vi "E709_All_VIs.vi"   [LabVIEW 2014, in "PiFOC.lvlib"]
doc: "This VI contains all high level and low level VIs valid for E-709. \nSee diagram for a survey of all E-709 high level and low level VIs. \nMenu / Browse / Show VI Hierarchy will show the file paths of the VIs. \nGlobal Variables are shown as Control as well as Indicator."
uses:
  PiFOC.lvlib
  Low Level/General command.llb/Controller names.ctl
  Low Level/Communication.llb/Available DLL interfaces.ctl
  Low Level/Communication.llb/Available DLLs.ctl
  Low Level/Communication.llb/Available interfaces.ctl
  Low Level/Communication.llb/Termination character.ctl
  Low Level/Analog control.llb/Available Analog Commands.ctl
  Low Level/Communication.llb/Global1.vi
  Low Level/General command.llb/Global2 (Array).vi
  Low Level/Communication.llb/Global DaisyChain.vi
  Low Level/Analog control.llb/Global Analog.vi
  Low Level/Support.llb/Unbunde/bundle interface clusters for PI Terminal.vi
panel:
  # "E-709 PI GCS LabVIEW driver set"
  # "This VI contains all high level and low level VIs valid for E-709. See diagram for a survey of all E-709 high \nlevel and low level VIs. Menu / Browse / Show VI Hierarchy will show the file paths of the VIs. Global \nVariables are shown as Control as well as Indicator."
types:
  T1 = typedef "PiFOC.lvlib/Available Analog Commands.ctl" = enum16{"INITIALIZE", "VOL?", "VOL ", "CLOSE", "MOV", "POS?", "VCO", "VCO?", "WAIT_WF", "TMN?", "TMX?", "VEL", "VEL?", "SAI?", "MVR", "ERR?", "#24", "STP", "*IDN?", "#5", "STE", "DRR?", "W_Wave", "HLP?", "W/R_Wave"}
  T2 = typedef "PiFOC.lvlib/Termination character.ctl" = enum16{"LF", "CR", "LFCR", "CRLF"}
  T3 = typedef "PiFOC.lvlib/Available interfaces.ctl" = u16
  T4 = typedef "PiFOC.lvlib/Available DLLs.ctl" = u16
  T5 = typedef "PiFOC.lvlib/Available DLL interfaces.ctl" = u16
  T6 = typedef "PiFOC.lvlib/Controller names.ctl" = enum16{"None", "Analog", "C-702", "C-843", "C-843.PM", "C-844", "C-848", "C-865", "C-866", "C-867", "C-880", "C-884", "E-516", "E-517", "E-709", "E-710", "E-712", "E-725", "E-753", "E-755", "E-761", "E-816", "E-861", "E-870", "E-871", "F-206", "HydraPollux", "M-840", "M-850", "M-8X0", "Mercury", "Mercury_GCS"}
  T7 = cluster{"Conversion factor":dbl[], "Velocity":dbl[], "Velocity control mode":bool, "AO.Resolution":dbl, "Lower voltage limit (V)":dbl, "Upper voltage limit (V)":dbl, "AO_WF_T (s)":dbl, "AI Sample Rate":dbl, "AI Samples/Channel":i32, "Hyperbit":bool, "Offset (V)":dbl[], "Hyperbit StayOnPos":bool, "Gain (V)":dbl[], "Bit rate (Hz)":dbl, "PWM rate (Hz)":dbl, "HyperBit Password":string, "AO.MaxRate":dbl, "Conversion offset":dbl[]}[]
  T8 = cluster{"No. of devices":i32, "Port ID":i32, "Devices":string[], "Description":string}[]
  T9 = cluster{"Conn. axes":string[], "Controller name":T6}[]
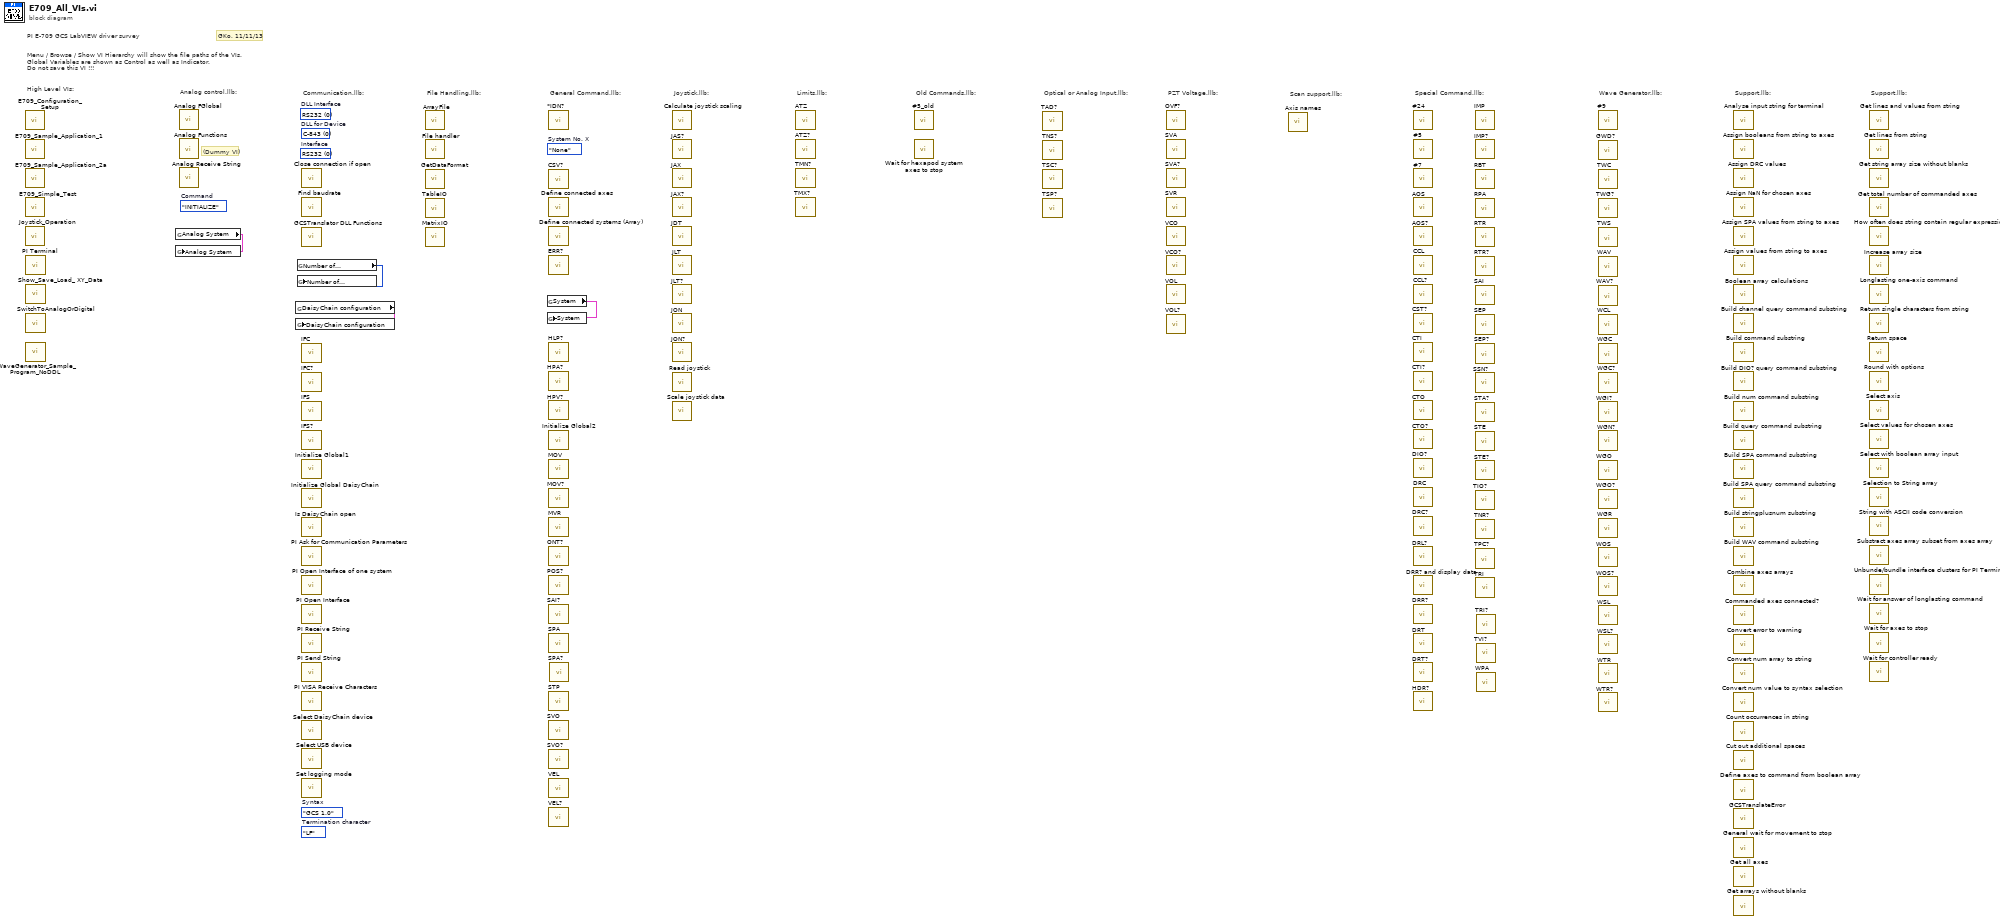
[diagram p0: block diagram]
diagram:
  (unwired) Available_Analog_Commands."INITIALIZE"  # Command
  (unwired) Termination_character."LF"  # Termination character
  (unwired) enum16{"GCS 1.0", "GCS 2.0"}."GCS 1.0"  # Syntax
  (unwired) T3 0 items=["RS232", "GPIB", "DLL", "TCP-IP"]  # Interface
  (unwired) T4 0 items=["C-843", "C-844", "E-710", "C-843.PM", "C-865", "E-761", "Mercury"]  # DLL for Device
  (unwired) T5 0 items=["RS232", "GPIB", "Board", "TCP-IP", "USB"]  # DLL Interface
  (unwired) Controller_names."None"  # System No. X
  # "Scan support.llb:"
  # "(Dummy VI)"
  # "GKo, 11/11/13"
  # "High Level VIs:"
  # "Analog control.llb:"
  # "Support.llb:"
  # "Wave Generator.llb:"
  # "Support.llb:"
  # "Special Command.llb:"
  # "PZT Voltage.llb:"
  # "Optical or Analog Input.llb:"
  # "Old Commands.llb:"
  # "Limits.llb:"
  # "Joystick.llb:"
  # "General Command.llb:"
  # "File Handling.llb:"
  # "Menu / Browse / Show VI Hierarchy will show the file paths of the VIs. \nGlobal Variables are shown as Control as well as Indicator.\nDo not save this VI !!!"
  # "PI E-709 GCS LabVIEW driver survey"
  # "Communication.llb:"
  n1 = call "E709_Configuration_Setup.vi"() -> ()  [unwired: 14 in, 6 out]
  n2 = call "E709_Sample_Application_1.vi"() -> ()  [unwired: 20 out]
  n3 = call "E709_Sample_Application_2a.vi"() -> ()  [unwired: 1 in, 15 out]
  n4 = call "E709_Simple_Test.vi"() -> ()  [unwired: 20 out]
  n5 = call "Joystick_Operation.vi"() -> ()  [unwired: 15 in, 5 out]
  n6 = call "PI Terminal.vi"() -> ()  [unwired: 20 out]
  n7 = call "Show_Save_Load_ XY_Data.vi"() -> ()  [unwired: 7 in, 13 out]
  n8 = call "SwitchToAnalogOrDigital.vi"() -> ()  [unwired: 9 in, 11 out]
  n9 = call "WaveGenerator_Sample_Program_NoDDL.vi"() -> ()  [unwired: 8 in, 12 out]
  n10 = global read "Global Analog.vi" "Analog System"() -> (w1:T7)
  n11 = global write "Global Analog.vi" "Analog System"(w1) -> ()
  n12 = call "Analog FGlobal.vi"() -> ()  [unwired: 3 in, 17 out]
  n13 = call "Analog Functions.vi"() -> ()  [unwired: 7 in, 13 out]
  n14 = call "Analog Receive String.vi"() -> ()  [unwired: 5 in, 15 out]
  n15 = global read "Global DaisyChain.vi" "DaisyChain configuration"() -> (w2:T8)
  n16 = global write "Global DaisyChain.vi" "DaisyChain configuration"(w2) -> ()
  n17 = global read "Global1.vi" "Number of\nsystems"() -> (w4:i32)
  n18 = global write "Global1.vi" "Number of\nsystems"(w4) -> ()
  n19 = call "Close connection if open.vi"() -> ()  [unwired: 3 in, 17 out]
  n20 = call "Find baudrate.vi"() -> ()  [unwired: 10 in, 10 out]
  n21 = call "GCSTranslator DLL Functions.vi"() -> ()  [unwired: 7 in, 13 out]
  n22 = call "IFC.vi"() -> ()  [unwired: 4 in, 16 out]
  n23 = call "IFC?.vi"() -> ()  [unwired: 4 in, 16 out]
  n24 = call "IFS.vi"() -> ()  [unwired: 5 in, 15 out]
  n25 = call "IFS?.vi"() -> ()  [unwired: 4 in, 16 out]
  n26 = call "Initialize Global1.vi"() -> ()  [unwired: 2 in, 18 out]
  n27 = call "Initialize Global DaisyChain.vi"() -> ()  [unwired: 2 in, 18 out]
  n28 = call "Is DaisyChain open.vi"() -> ()  [unwired: 2 in, 18 out]
  n29 = call "PI Ask for Communication Parameters.vi"() -> ()  [unwired: 20 out]
  n30 = call "PI Open Interface of one system.vi"() -> ()  [unwired: 12 in, 8 out]
  n31 = call "PI Open Interface.vi"() -> ()  [unwired: 12 in, 8 out]
  n32 = call "PI Receive String.vi"() -> ()  [unwired: 3 in, 17 out]
  n33 = call "PI Send String.vi"() -> ()  [unwired: 4 in, 16 out]
  n34 = call "PI VISA Receive Characters.vi"() -> ()  [unwired: 3 in, 17 out]
  n35 = call "Select DaisyChain device.vi"() -> ()  [unwired: 9 in, 11 out]
  n36 = call "Select USB device.vi"() -> ()  [unwired: 5 in, 15 out]
  n37 = call "Set logging mode.vi"() -> ()  [unwired: 4 in, 16 out]
  n38 = call "ArrayFile.vi"() -> ()  [unwired: 20 out]
  n39 = call "File handler.vi"() -> ()  [unwired: 6 in, 14 out]
  n40 = call "GetDataFormat.vi"() -> ()  [unwired: 2 in, 18 out]
  n41 = call "TableIO.vi"() -> ()  [unwired: 6 in, 14 out]
  n42 = call "MatrixIO.vi"() -> ()  [unwired: 7 in, 13 out]
  n43 = global read "Global2 (Array).vi" "System"() -> (w3:T9)
  n44 = global write "Global2 (Array).vi" "System"(w3) -> ()
  n45 = call "*IDN?.vi"() -> ()  [unwired: 2 in, 18 out]
  n46 = call "CSV?.vi"() -> ()  [unwired: 2 in, 18 out]
  n47 = call "Define connected axes.vi"() -> ()  [unwired: 5 in, 15 out]
  n48 = call "Define connected systems (Array).vi"() -> ()  [unwired: 4 in, 16 out]
  n49 = call "ERR?.vi"() -> ()  [unwired: 2 in, 18 out]
  n50 = call "HLP?.vi"() -> ()  [unwired: 2 in, 18 out]
  n51 = call "HPA?.vi"() -> ()  [unwired: 2 in, 18 out]
  n52 = call "HPV?.vi"() -> ()  [unwired: 2 in, 18 out]
  n53 = call "Initialize Global2.vi"() -> ()  [unwired: 2 in, 18 out]
  n54 = call "MOV.vi"() -> ()  [unwired: 5 in, 15 out]
  n55 = call "MOV?.vi"() -> ()  [unwired: 5 in, 15 out]
  n56 = call "MVR.vi"() -> ()  [unwired: 5 in, 15 out]
  n57 = call "ONT?.vi"() -> ()  [unwired: 5 in, 15 out]
  n58 = call "POS?.vi"() -> ()  [unwired: 5 in, 15 out]
  n59 = call "SAI?.vi"() -> ()  [unwired: 5 in, 15 out]
  n60 = call "SPA.vi"() -> ()  [unwired: 10 in, 10 out]
  n61 = call "STP.vi"() -> ()  [unwired: 5 in, 15 out]
  n62 = call "SVO.vi"() -> ()  [unwired: 5 in, 15 out]
  n63 = call "SVO?.vi"() -> ()  [unwired: 5 in, 15 out]
  n64 = call "VEL.vi"() -> ()  [unwired: 6 in, 14 out]
  n65 = call "VEL?.vi"() -> ()  [unwired: 5 in, 15 out]
  n66 = call "SPA?.vi"() -> ()  [unwired: 7 in, 13 out]
  n67 = call "Calculate joystick scaling.vi"() -> ()  [unwired: 6 in, 14 out]
  n68 = call "JAS?.vi"() -> ()  [unwired: 5 in, 15 out]
  n69 = call "JAX.vi"() -> ()  [unwired: 5 in, 15 out]
  n70 = call "JAX?.vi"() -> ()  [unwired: 5 in, 15 out]
  n71 = call "JDT.vi"() -> ()  [unwired: 5 in, 15 out]
  n72 = call "JLT.vi"() -> ()  [unwired: 7 in, 13 out]
  n73 = call "JLT?.vi"() -> ()  [unwired: 7 in, 13 out]
  n74 = call "JON.vi"() -> ()  [unwired: 4 in, 16 out]
  n75 = call "JON?.vi"() -> ()  [unwired: 4 in, 16 out]
  n76 = call "Read joystick.vi"() -> ()  [unwired: 2 in, 18 out]
  n77 = call "Scale joystick data.vi"() -> ()  [unwired: 8 in, 12 out]
  n78 = call "ATZ.vi"() -> ()  [unwired: 6 in, 14 out]
  n79 = call "ATZ?.vi"() -> ()  [unwired: 5 in, 15 out]
  n80 = call "TMN?.vi"() -> ()  [unwired: 5 in, 15 out]
  n81 = call "TMX?.vi"() -> ()  [unwired: 5 in, 15 out]
  n82 = call "#5_old.vi"() -> ()  [unwired: 2 in, 18 out]
  n83 = call "Wait for hexapod system axes to stop.vi"() -> ()  [unwired: 5 in, 15 out]
  n84 = call "TAD?.vi"() -> ()  [unwired: 5 in, 15 out]
  n85 = call "TNS?.vi"() -> ()  [unwired: 5 in, 15 out]
  n86 = call "TSC?.vi"() -> ()  [unwired: 2 in, 18 out]
  n87 = call "TSP?.vi"() -> ()  [unwired: 5 in, 15 out]
  n88 = call "OVF?.vi"() -> ()  [unwired: 5 in, 15 out]
  n89 = call "SVA.vi"() -> ()  [unwired: 5 in, 15 out]
  n90 = call "SVA?.vi"() -> ()  [unwired: 5 in, 15 out]
  n91 = call "SVR.vi"() -> ()  [unwired: 5 in, 15 out]
  n92 = call "VCO.vi"() -> ()  [unwired: 4 in, 16 out]
  n93 = call "VCO?.vi"() -> ()  [unwired: 5 in, 15 out]
  n94 = call "VOL.vi"() -> ()  [unwired: 5 in, 15 out]
  n95 = call "VOL?.vi"() -> ()  [unwired: 5 in, 15 out]
  n96 = call "Axis names.vi"() -> ()  [unwired: 1 in, 19 out]
  n97 = call "#24.vi"() -> ()  [unwired: 2 in, 18 out]
  n98 = call "#5.vi"() -> ()  [unwired: 2 in, 18 out]
  n99 = call "#7.vi"() -> ()  [unwired: 2 in, 18 out]
  n100 = call "AOS.vi"() -> ()  [unwired: 5 in, 15 out]
  n101 = call "AOS?.vi"() -> ()  [unwired: 5 in, 15 out]
  n102 = call "CCL.vi"() -> ()  [unwired: 4 in, 16 out]
  n103 = call "CCL?.vi"() -> ()  [unwired: 2 in, 18 out]
  n104 = call "CST?.vi"() -> ()  [unwired: 5 in, 15 out]
  n105 = call "CTI.vi"() -> ()  [unwired: 6 in, 14 out]
  n106 = call "CTI?.vi"() -> ()  [unwired: 5 in, 15 out]
  n107 = call "CTO.vi"() -> ()  [unwired: 6 in, 14 out]
  n108 = call "CTO?.vi"() -> ()  [unwired: 5 in, 15 out]
  n109 = call "DIO?.vi"() -> ()  [unwired: 6 in, 14 out]
  n110 = call "DRC.vi"() -> ()  [unwired: 6 in, 14 out]
  n111 = call "DRC?.vi"() -> ()  [unwired: 4 in, 16 out]
  n112 = call "DRL?.vi"() -> ()  [unwired: 4 in, 16 out]
  n113 = call "DRR? and display data.vi"() -> ()  [unwired: 7 in, 13 out]
  n114 = call "DRR?.vi"() -> ()  [unwired: 8 in, 12 out]
  n115 = call "DRT.vi"() -> ()  [unwired: 5 in, 15 out]
  n116 = call "DRT?.vi"() -> ()  [unwired: 4 in, 16 out]
  n117 = call "HDR?.vi"() -> ()  [unwired: 3 in, 17 out]
  n118 = call "IMP.vi"() -> ()  [unwired: 5 in, 15 out]
  n119 = call "IMP?.vi"() -> ()  [unwired: 6 in, 14 out]
  n120 = call "RBT.vi"() -> ()  [unwired: 2 in, 18 out]
  n121 = call "RPA.vi"() -> ()  [unwired: 6 in, 14 out]
  n122 = call "RTR.vi"() -> ()  [unwired: 3 in, 17 out]
  n123 = call "RTR?.vi"() -> ()  [unwired: 2 in, 18 out]
  n124 = call "SAI.vi"() -> ()  [unwired: 4 in, 16 out]
  n125 = call "SEP.vi"() -> ()  [unwired: 11 in, 9 out]
  n126 = call "SEP?.vi"() -> ()  [unwired: 7 in, 13 out]
  n127 = call "SSN?.vi"() -> ()  [unwired: 4 in, 16 out]
  n128 = call "STA?.vi"() -> ()  [unwired: 5 in, 15 out]
  n129 = call "STE.vi"() -> ()  [unwired: 6 in, 14 out]
  n130 = call "STE?.vi"() -> ()  [unwired: 6 in, 14 out]
  n131 = call "TIO?.vi"() -> ()  [unwired: 2 in, 18 out]
  n132 = call "TNR?.vi"() -> ()  [unwired: 2 in, 18 out]
  n133 = call "TPC?.vi"() -> ()  [unwired: 2 in, 18 out]
  n134 = call "TRI.vi"() -> ()  [unwired: 4 in, 16 out]
  n135 = call "TRI?.vi"() -> ()  [unwired: 4 in, 16 out]
  n136 = call "TVI?.vi"() -> ()  [unwired: 3 in, 17 out]
  n137 = call "WPA.vi"() -> ()  [unwired: 7 in, 13 out]
  n138 = call "#9.vi"() -> ()  [unwired: 2 in, 18 out]
  n139 = call "GWD?.vi"() -> ()  [unwired: 6 in, 14 out]
  n140 = call "TWC.vi"() -> ()  [unwired: 2 in, 18 out]
  n141 = call "TWG?.vi"() -> ()  [unwired: 2 in, 18 out]
  n142 = call "TWS.vi"() -> ()  [unwired: 5 in, 15 out]
  n143 = call "WAV.vi"() -> ()  [unwired: 19 in, 9 out]
  n144 = call "WAV?.vi"() -> ()  [unwired: 4 in, 16 out]
  n145 = call "WCL.vi"() -> ()  [unwired: 5 in, 15 out]
  n146 = call "WGC.vi"() -> ()  [unwired: 4 in, 16 out]
  n147 = call "WGC?.vi"() -> ()  [unwired: 5 in, 15 out]
  n148 = call "WGO.vi"() -> ()  [unwired: 4 in, 16 out]
  n149 = call "WGO?.vi"() -> ()  [unwired: 5 in, 15 out]
  n150 = call "WGR.vi"() -> ()  [unwired: 2 in, 18 out]
  n151 = call "WOS.vi"() -> ()  [unwired: 5 in, 15 out]
  n152 = call "WOS?.vi"() -> ()  [unwired: 4 in, 16 out]
  n153 = call "WSL.vi"() -> ()  [unwired: 4 in, 16 out]
  n154 = call "WSL?.vi"() -> ()  [unwired: 4 in, 16 out]
  n155 = call "WTR.vi"() -> ()  [unwired: 5 in, 15 out]
  n156 = call "WTR?.vi"() -> ()  [unwired: 4 in, 16 out]
  n157 = call "WGI?.vi"() -> ()  [unwired: 5 in, 15 out]
  n158 = call "WGN?.vi"() -> ()  [unwired: 5 in, 15 out]
  n159 = call "Analyse input string for terminal.vi"() -> ()  [unwired: 2 in, 18 out]
  n160 = call "Assign booleans from string to axes.vi"() -> ()  [unwired: 5 in, 15 out]
  n161 = call "Assign DRC values.vi"() -> ()  [unwired: 3 in, 17 out]
  n162 = call "Assign NaN for chosen axes.vi"() -> ()  [unwired: 4 in, 16 out]
  n163 = call "Assign SPA values from string to axes.vi"() -> ()  [unwired: 7 in, 13 out]
  n164 = call "Assign values from string to axes.vi"() -> ()  [unwired: 6 in, 14 out]
  n165 = call "Boolean array calculations.vi"() -> ()  [unwired: 4 in, 16 out]
  n166 = call "Build channel query command substring.vi"() -> ()  [unwired: 7 in, 13 out]
  n167 = call "Build command substring.vi"() -> ()  [unwired: 7 in, 13 out]
  n168 = call "Build DIO? query command substring.vi"() -> ()  [unwired: 6 in, 14 out]
  n169 = call "Build num command substring.vi"() -> ()  [unwired: 3 in, 17 out]
  n170 = call "Build query command substring.vi"() -> ()  [unwired: 5 in, 15 out]
  n171 = call "Build SPA command substring.vi"() -> ()  [unwired: 10 in, 10 out]
  n172 = call "Build SPA query command substring.vi"() -> ()  [unwired: 5 in, 15 out]
  n173 = call "Build stringplusnum substring.vi"() -> ()  [unwired: 10 in, 10 out]
  n174 = call "Build WAV command substring.vi"() -> ()  [unwired: 18 in, 10 out]
  n175 = call "Combine axes arrays.vi"() -> ()  [unwired: 2 in, 18 out]
  n176 = call "Commanded axes connected?.vi"() -> ()  [unwired: 3 in, 17 out]
  n177 = call "Convert error to warning.vi"() -> ()  [unwired: 2 in, 18 out]
  n178 = call "Convert num array to string.vi"() -> ()  [unwired: 2 in, 18 out]
  n179 = call "Convert num value to syntax selection.vi"() -> ()  [unwired: 1 in, 19 out]
  n180 = call "Count occurrences in string.vi"() -> ()  [unwired: 2 in, 18 out]
  n181 = call "Cut out additional spaces.vi"() -> ()  [unwired: 2 in, 18 out]
  n182 = call "Define axes to command from boolean array.vi"() -> ()  [unwired: 4 in, 16 out]
  n183 = call "GCSTranslateError.vi"() -> ()  [unwired: 1 in, 19 out]
  n184 = call "General wait for movement to stop.vi"() -> ()  [unwired: 8 in, 12 out]
  n185 = call "Get all axes.vi"() -> ()  [unwired: 1 in, 19 out]
  n186 = call "Get arrays without blanks.vi"() -> ()  [unwired: 3 in, 17 out]
  n187 = call "Get lines and values from string.vi"() -> ()  [unwired: 2 in, 18 out]
  n188 = call "Get lines from string.vi"() -> ()  [unwired: 3 in, 17 out]
  n189 = call "Get string array size without blanks.vi"() -> ()  [unwired: 1 in, 19 out]
  n190 = call "Get total number of commanded axes.vi"() -> ()  [unwired: 2 in, 18 out]
  n191 = call "How often does string contain regular expression?.vi"() -> ()  [unwired: 2 in, 18 out]
  n192 = call "Increase array size.vi"() -> ()  [unwired: 3 in, 17 out]
  n193 = call "Longlasting one-axis command.vi"() -> ()  [unwired: 7 in, 13 out]
  n194 = call "Return single characters from string.vi"() -> ()  [unwired: 3 in, 17 out]
  n195 = call "Return space.vi"() -> ()  [unwired: 2 in, 18 out]
  n196 = call "Round with options.vi"() -> ()  [unwired: 4 in, 16 out]
  n197 = call "Select axis.vi"() -> ()  [unwired: 2 in, 18 out]
  n198 = call "Select values for chosen axes.vi"() -> ()  [unwired: 5 in, 15 out]
  n199 = call "Select with boolean array input.vi"() -> ()  [unwired: 4 in, 16 out]
  n200 = call "Selection to String array.vi"() -> ()  [unwired: 2 in, 18 out]
  n201 = call "String with ASCII code conversion.vi"() -> ()  [unwired: 1 in, 19 out]
  n202 = call "Substract axes array subset from axes array.vi"() -> ()  [unwired: 2 in, 18 out]
  n203 = call "Unbunde/bundle interface clusters for PI Terminal.vi"() -> ()  [unwired: 6 in, 14 out]
  n204 = call "Wait for answer of longlasting command.vi"() -> ()  [unwired: 3 in, 17 out]
  n205 = call "Wait for axes to stop.vi"() -> ()  [unwired: 7 in, 13 out]
  n206 = call "Wait for controller ready.vi"() -> ()  [unwired: 4 in, 16 out]
